vi "Read Counter Value.vi"(8 "error in (no error)":errorcluster, 11 "VISA resource name":refnum<visa-resource-name>) -> (0 "error out":errorcluster, 2 "Count":i32, 3 "VISA resource name out":refnum<visa-resource-name>)   [LabVIEW 2020, in "BDAQ-6104.lvlib"]
doc: "Starts the edge counter."
uses:
  <instrlib>/BDAQ-6104/BDAQ-6104.lvlib
panel:
  out "read buffer":string
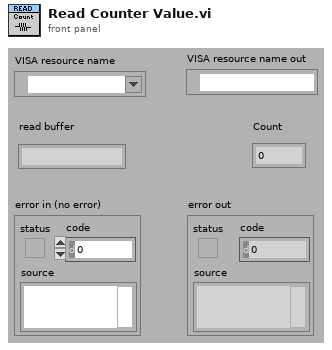
[diagram p1: front panel]
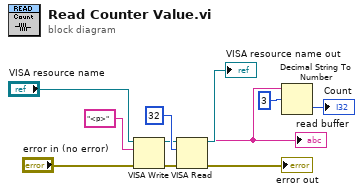
[diagram p0: block diagram]
diagram:
  n1 = VISA Write(VISA resource name="VISA resource name", write buffer="<p>" ("command"), error in (no error)="error in (no error)") -> (VISA resource name out=w6:refnum<visa-resource-name>, error out=w8:errorcluster)  [unwired: 1 out]
  n2 = VISA Read(VISA resource name=w6, byte count=u32 32, error in (no error)=w8) -> (VISA resource name out=→"VISA resource name out":refnum<visa-resource-name>, read buffer=w3:string, error out=→"error out":errorcluster)  [unwired: 1 out]
  "read buffer" <- w3
  n3 = Decimal String To Number(string=w3, offset=3) -> (number=→"Count":i32)  [unwired: 1 in, 1 out]
